vi "Fct_Limite_Température.vi"(11 "Température":dbl) -> (3 "Booléen":bool)   [LabVIEW 2017]
panel:
  out "Motif":string
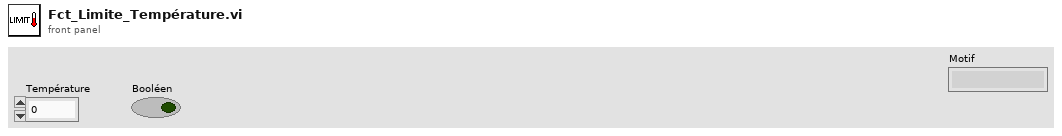
[diagram p1: front panel]
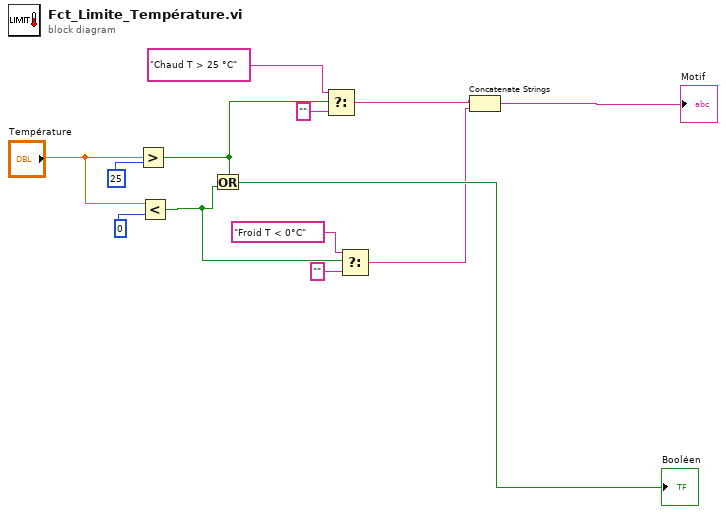
[diagram p0: block diagram]
diagram:
  n1 = Greater?(x="Température", y=25) -> (0:w9:bool)
  n2 = Less?(x="Température", y=0) -> (x < y?=w8:bool)
  n3 = Or(x=w9, y=w8) -> (x .or. y?=→"Booléen":bool)
  n4 = Select(t="Chaud T > 25 °C", s=w9, f="" ("cas faux")) -> (s? t:f=w3:string)
  n5 = Select(t="Froid T < 0°C", s=w8, f="" ("cas faux")) -> (s? t:f=w2:string)
  n6 = Concatenate Strings(w3, w2) -> (→"Motif":string)
